vi "APS spiral ca all.vi"(0 "Axis_ID_Array":i32, 1 "Option":i32, 2 "CenterArray":dbl, 3 "NormalArray":dbl, 4 "Angle":dbl, 5 "DeltaH":dbl, 6 "FinalR":dbl, 7 "error in (no error)":errorcluster caption="错误输入（无错误）", 8 "TransPara":dbl, 9 "Vs":dbl, 10 "Vm":dbl, 11 "Ve":dbl, 12 "Acc":dbl, 13 "Dec":dbl, 14 "SFac":dbl, 15 "Wait":cluster{"h_event":u32, "i32_ret":i32}) -> (18 "TransPara out":dbl, 20 "Axis_ID_Array out":i32, 21 "Wait out":cluster{"h_event":u32, "i32_ret":i32}, 22 "CenterArray out":dbl, 23 "NormalArray out":dbl, 24 "function return":i32, 27 "error out":errorcluster caption="错误输出")   [LabVIEW 2011, in "APS168.lvlib"]
doc: "I32 FNTYPE APS_spiral_ca_all( I32 *Axis_ID_Array, I32 Option, F64 *CenterArray, F64 *NormalArray, F64 Angle, F64 DeltaH, F64 FinalR, F64 *TransPara, F64 Vs, F64 Vm, F64 Ve, F64 Acc,F64 Dec, F64 SFac, ASYNCALL *Wait );"
uses:
  APS168.lvlib
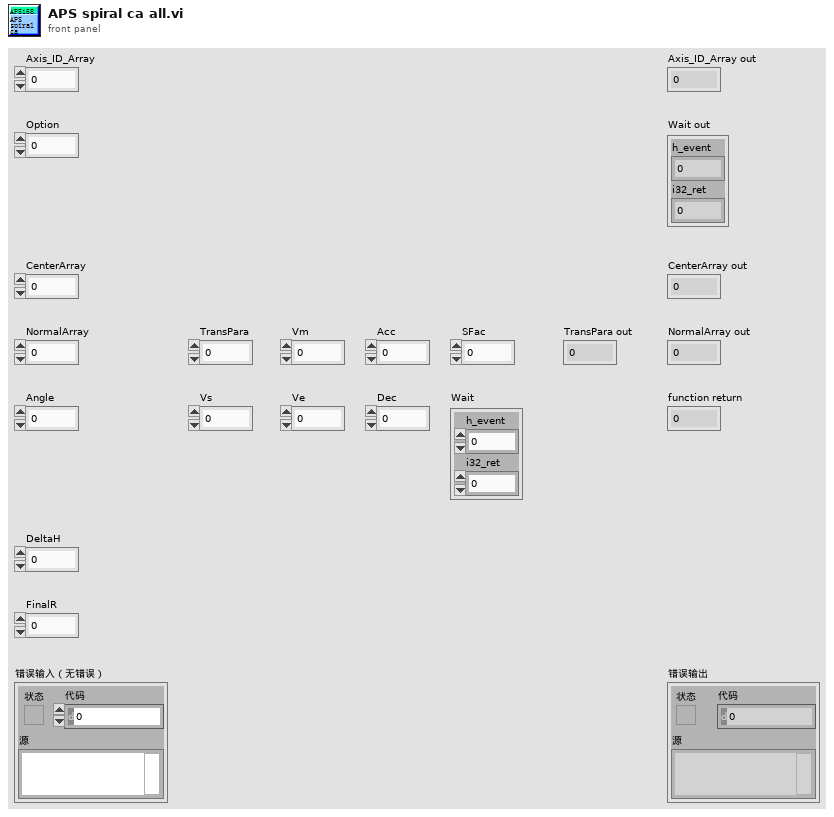
[diagram p1: front panel]
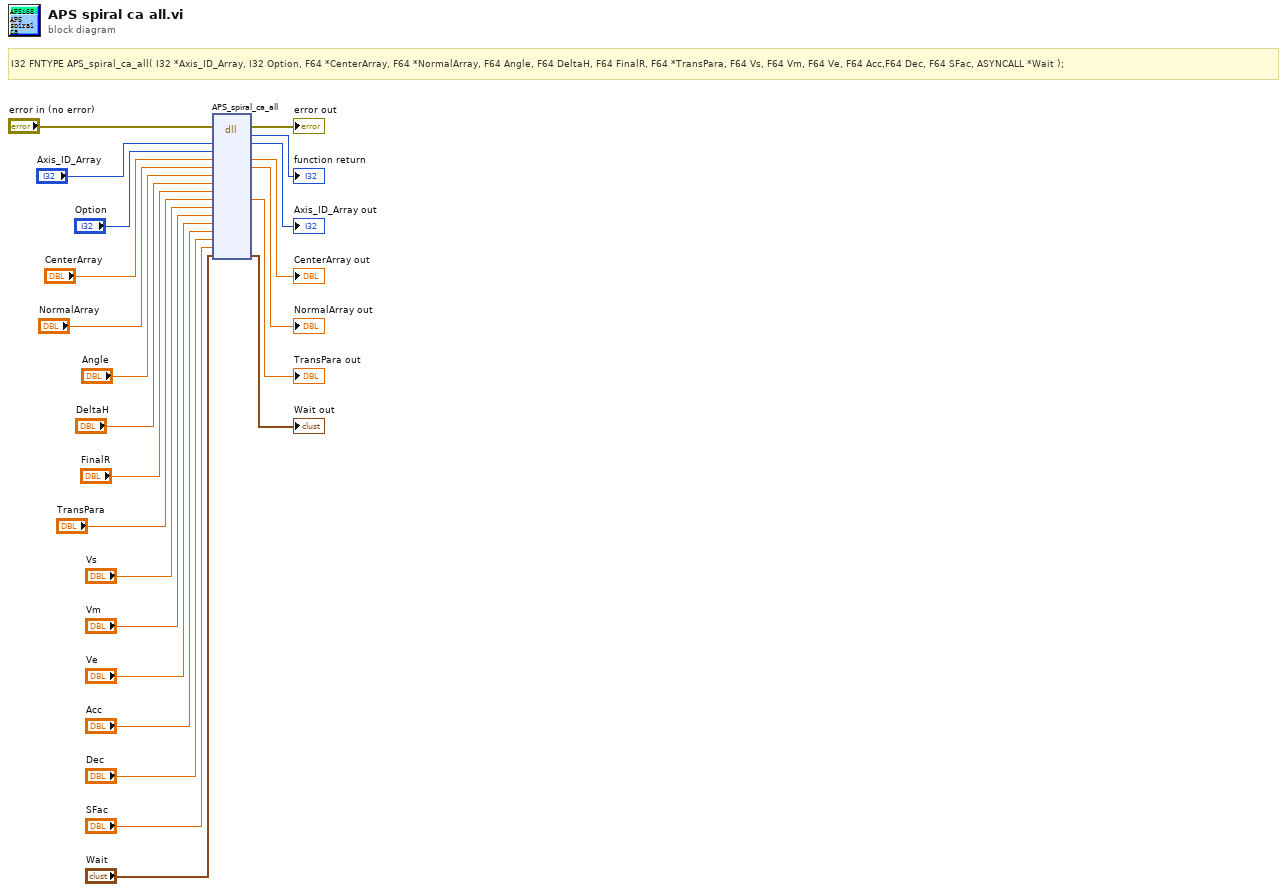
[diagram p0: block diagram]
diagram:
  # "I32 FNTYPE APS_spiral_ca_all( I32 *Axis_ID_Array, I32 Option, F64 *CenterArray, F64 *NormalArray, F64 Angle, F64 DeltaH, F64 FinalR, F64 *TransPara, F64 Vs, F64 Vm, F64 Ve, F64 Acc,F64 Dec, F64 SFac, ASYNCALL *Wait );"
  n1 = dll-call lib="PTH1Labs E软件ADLINK 204CAPS_1_7_1_LIB line 连续运动204APS168.*" fn="APS_spiral_ca_all"(error in="error in (no error)", "Axis_ID_Array"="Axis_ID_Array", "Option"="Option", "CenterArray"="CenterArray", "NormalArray"="NormalArray", "Angle"="Angle", "DeltaH"="DeltaH", "FinalR"="FinalR", "TransPara"="TransPara", "Vs"="Vs", "Vm"="Vm", "Ve"="Ve", "Acc"="Acc", "Dec"="Dec", "SFac"="SFac", "Wait"="Wait") -> (error out=→"error out":errorcluster, →"function return":i32, "Axis_ID_Array"=→"Axis_ID_Array out":i32, "CenterArray"=→"CenterArray out":dbl, "NormalArray"=→"NormalArray out":dbl, "TransPara"=→"TransPara out":dbl, "Wait"=→"Wait out":cluster{"h_event":u32, "i32_ret":i32})  [unwired: 12 in, 1 out]
